vi "Create Sysdef Tree from DB Channel Clusters_RTs_Create MCs.vi"(5 "modeCodes":T4[](array[typedef]), 6 "Autocreate Rx timestamp chans?":bool, 7 "messageBuffers":T2(array[cluster]), 8 "error in (no error)":errorcluster, 10 "rtMode":T3, 11 "Section Ptr in":T1 format="%.0x") -> (0 "error out":errorcluster)   [LabVIEW 2017, in "Ballard 1553 System Explorer.lvlib"]
uses:
  Ballard 1553 System Explorer.lvlib
  <vilib>/NI Veristand/Custom Device API/Custom Device Item Ref.ctl
  Parse XML Ballard/Ballard_RT modeCode.ctl
  Parse XML Ballard/Ballard_RT direction.ctl
  Parse XML Ballard/Ballard_RT rtMode.ctl
  <vilib>/NI Veristand/Custom Device API/Custom Device Channel Type.ctl
  <vilib>/NI Veristand/Custom Device API/Custom Device Channel.ctl
  Shared/Controls and Global/Global.vi
  <vilib>/NI Veristand/Custom Device API/Set Item Property (I32).vi
  <vilib>/NI Veristand/Custom Device API/Set Item Property (U16).vi
  <vilib>/NI VeriStand/Custom Device API/Custom Device API.lvlib
  Shared/Ballard 1553 Shared.lvlib
panel:
  out "Section Ptr out":T1 format="%.0x"
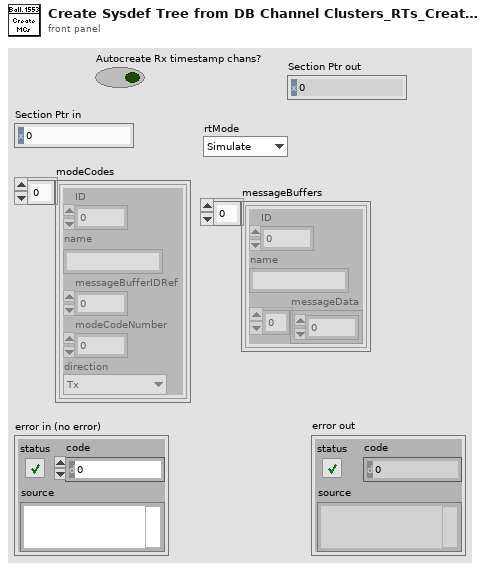
[diagram p1: front panel]
types:
  T1 = typedef "Custom Device API.lvlib/Custom Device Item Ref.ctl" = u64
  T2 = cluster{"ID":i32, "name":string, "messageData":u16[]}[]
  T3 = typedef "Ballard 1553 System Explorer.lvlib/Ballard_RT rtMode.ctl" = enum16{"Simulate", "Monitor", "Disable"}
  T4 = typedef "Ballard 1553 System Explorer.lvlib/Ballard_RT modeCode.ctl" = cluster{"ID":i32, "name":string, "messageBufferIDRef":i32, "modeCodeNumber":i8, "direction":T5}
  T5 = typedef "Ballard 1553 System Explorer.lvlib/Ballard_RT direction.ctl" = enum16{"Tx", "Rx"}
  T6 = typedef "Custom Device API.lvlib/Custom Device Channel Type.ctl" = enum16{"Input", "Output"}
  T7 = typedef "Custom Device API.lvlib/Custom Device Channel.ctl" = cluster{"Type":T6, "Units":string, "Default Value":dbl, "Faultable":bool, "Scalable":bool}
  T8 = enum16{"DW", "STC", "SPC", "SW", "TI MC", "AC", "TI WC"}
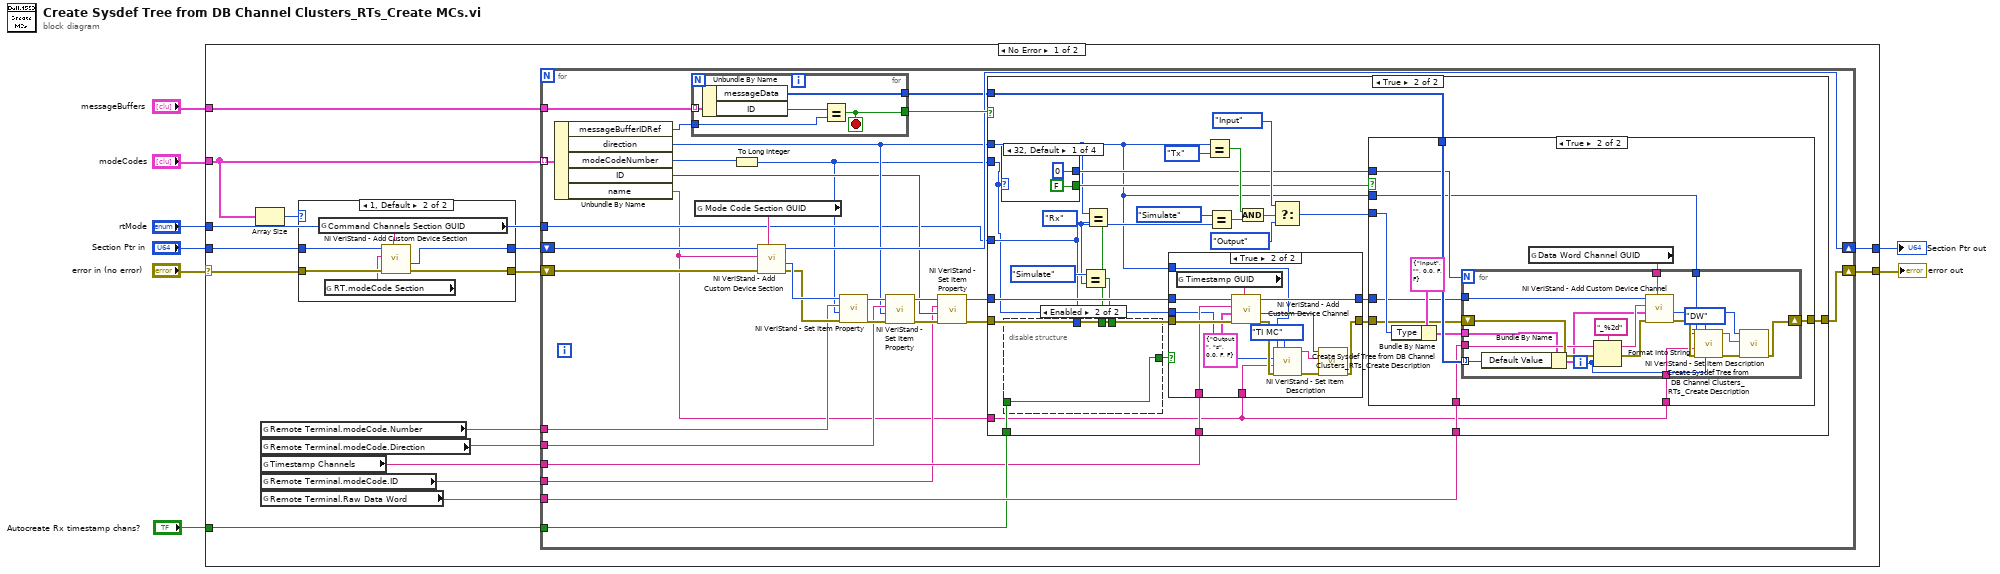
[diagram p0: block diagram]
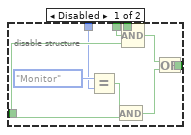
[diagram p3: hidden frame]
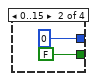
[diagram p4: hidden frame]
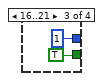
[diagram p5: hidden frame]
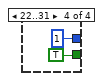
[diagram p6: hidden frame]
diagram:
  n1 = case shown="No Error" "error in (no error)" {
    selector: "error in (no error)" -> [w12 w165]
    tunnel: [w24 w164] -> w8
    tunnel: [w23 w165] -> w2
    tunnel: "modeCodes" -> [w14 _]
    tunnel: "Autocreate Rx timestamp chans?" -> [w21 _]
    tunnel: "messageBuffers" -> [w20 _]
    tunnel: "Section Ptr in" -> [w13 w164]
    tunnel: "rtMode" -> [w16 _]
    frame No Error {
      n2 = Array Size(array=w14) -> (size(s)=w15:i32)
      n3 = global read "Global.vi" "Remote Terminal.modeCode.Number"() -> (w17:string)
      n4 = global read "Global.vi" "Remote Terminal.modeCode.Direction"() -> (w18:string)
      n5 = global read "Global.vi" "Timestamp Channels"() -> (w22:string)
      n6 = global read "Global.vi" "Remote Terminal.modeCode.ID"() -> (w9:string)
      n7 = global read "Global.vi" "Remote Terminal.Raw Data Word"() -> (w19:string)
      n8 = case shown="1, Default" w15 {
        tunnel: w12 -> [w157 w162]
        tunnel: w13 -> [w156 w163]
        tunnel: [w157 w161] -> w10
        tunnel: [w156 w158] -> w11
        frame 0 {
        }
        frame 1, Default {
          n9 = global read "Global.vi" "Command Channels Section GUID"() -> (w160:string)
          n10 = global read "Global.vi" "RT.modeCode Section"() -> (w159:string)
          n11 = call <vilib>:"NI VeriStand - Add Custom Device Section.vi"("GUID (Default Section)"=w160, "error in (no error)"=w162, "Section Name"=w159, "Parent Ref in"=w163) -> ("error out"=w161:errorcluster, "Section Ptr"=w158:T1)  [unwired: 4 in, 2 out]
        }
      }
      n12 = for {
        tunnel: w14 -> [w54] mode=indexing
        shift-right: [w41] -> w23
        shift-left: w10 -> [w27]
        shift-right: [w42] -> w24
        shift-left: w11 -> [w53]
        tunnel: w17 -> [w50]
        tunnel: w18 -> [w47]
        tunnel: w19 -> [w39]
        tunnel: w20 -> [w45]
        tunnel: w21 -> [w38]
        tunnel: w22 -> [w37]
        tunnel: w9 -> [w29]
        tunnel: w16 -> [w28]
        n13 = Unbundle By Name(w54) -> ("messageBufferIDRef"=w44:i32, "direction"=w35:T5, "modeCodeNumber"=w36:i8, "ID"=w30:i32, "name"=w25:string)
        n14 = for {
          tunnel: w45 -> [w155] mode=indexing
          tunnel: w44 -> [w153]
          tunnel: [w152] -> w40
          tunnel: [w151] -> w43
          stop <- w151 stop-if-true
          n15 = Unbundle By Name(w155) -> ("messageData"=w152:u16[], "ID"=w154:i32)
          n16 = Equal?(x=w154, y=w153) -> (x = y?=w151:bool)
        }
        n17 = global read "Global.vi" "Mode Code Section GUID"() -> (w46:string)
        n18 = To Long Integer(number=w36) -> (32bit integer=w26:i32)
        n19 = call <vilib>:"NI VeriStand - Add Custom Device Section.vi"("GUID (Default Section)"=w46, "error in (no error)"=w27, "Section Name"=w25, "Parent Ref in"=w53) -> ("error out"=w51:errorcluster, "Section Ptr"=w52:T1, "Parent Ref out"=w42:T1)  [unwired: 4 in, 1 out]
        n20 = call-poly <vilib>:"NI VeriStand - Set Item Property.vi"("error in (no error)"=w51, "Value"=w26, "Property Name"=w50, "Item Ref in"=w52) -> ("error out"=w49:errorcluster, "Item Ref out"=w48:T1)  [unwired: 5 in, 1 out]
        n21 = call-poly <vilib>:"NI VeriStand - Set Item Property.vi"("error in (no error)"=w49, "Value"=w35, "Property Name"=w47, "Item Ref in"=w48) -> ("error out"=w33:errorcluster, "Item Ref out"=w34:T1)  [unwired: 5 in, 1 out]
        n22 = call-poly <vilib>:"NI VeriStand - Set Item Property.vi"("error in (no error)"=w33, "Value"=w30, "Property Name"=w29, "Item Ref in"=w34) -> ("error out"=w31:errorcluster, "Item Ref out"=w32:T1)  [unwired: 5 in, 1 out]
        n23 = case shown="True" w43 {
          tunnel: w31 -> [w55 w71]
          tunnel: w32 -> [_ w72]
          tunnel: [w55 w73] -> w41
          tunnel: w40 -> [_ w83]
          tunnel: w39 -> [_ w82]
          tunnel: w28 -> [_ w64]
          tunnel: w35 -> [_ w57]
          tunnel: w38 -> [_ w69]
          tunnel: w37 -> [_ w63]
          tunnel: w26 -> [_ w58]
          tunnel: w25 -> [_ w56]
          frame False {
          }
          frame True {
            n24 = case shown="32, Default" w58 {
              tunnel: [i8 0 ("Words (WC)") i8 0 ("Words (WC)") i8 1 ("Words (WC)") i8 1 ("Words (WC)")] -> w59
              tunnel: [FALSE ("2 Status Channels") FALSE ("2 Status Channels") TRUE ("2 Status Channels") TRUE ("2 Status Channels")] -> w60
              frame 32, Default {
              }
              frame 0..15 {
              }
              frame 16..21 {
              }
              frame 22..31 {
              }
            }
            n25 = Equal?(x=Ballard_RT_rtMode."Simulate", y=w64) -> (x = y?=w67:bool)
            n26 = Equal?(x=w57, y=Ballard_RT_direction."Rx") -> (x = y?=w65:bool)
            n27 = disable-structure shown="Enabled" {
              disable-tunnel: [w92 w93] -> w70
              disable-tunnel: w69 -> [w88 w93]
              disable-tunnel: w67 -> [w86 _]
              disable-tunnel: w65 -> [w85 _]
              disable-tunnel: w64 -> [w84 _]
              frame Disabled {
                n28 = Equal?(x=Ballard_RT_rtMode."Monitor", y=w84) -> (x = y?=w90:bool)
                n29 = And(x=w90, y=w88) -> (x .and. y?=w89:bool)
                n30 = Compound Arithmetic op=AND(w86, w85, w88) -> (w87:bool)
                n31 = Or(x=w87, y=w89) -> (x .or. y?=w92:bool)
              }
              frame Enabled {
              }
            }
            n32 = case shown="True" w70 {
              tunnel: w72 -> [w135 w150]
              tunnel: w71 -> [w134 w149]
              tunnel: [w135 w148] -> w61
              tunnel: [w134 w140] -> w62
              tunnel: w63 -> [_ w145]
              tunnel: w56 -> [_ w139]
              tunnel: w57 -> [_ w138]
              tunnel: w58 -> [_ w137]
              frame False {
              }
              frame True {
                n33 = global read "Global.vi" "Timestamp GUID"() -> (w147:string)
                n34 = call <vilib>:"NI VeriStand - Add Custom Device Channel.vi"("GUID (Default Channel)"=w147, "error in (no error)"=w149, "Channel"=T7 {"Type"=enum."Output", "Units"="s", "Default Value"=0.0, "Faultable"=FALSE, "Scalable"=FALSE}, "Channel Name"=w145, "Parent Ref in"=w150) -> ("error out"=w141:errorcluster, "Channel Ref"=w142:T1, "Parent Ref out"=w148:T1)  [unwired: 3 in, 1 out]
                n35 = call "Create Sysdef Tree from DB Channel Clusters_RTs_Create Description.vi"("Type"=T8."TI MC", "error in (no error)"=w141, "Name"=w139, "SA/MC"=w137, "Direction"=w138) -> ("error out"=w143:errorcluster, "Description (Out)"=w144:string)  [unwired: 5 in]
                n36 = call <vilib>:"NI VeriStand - Set Item Description.vi"("error in (no error)"=w143, "Description"=w144, "Item Ref in"=w142) -> ("error out"=w140:errorcluster)  [unwired: 6 in, 2 out]
              }
            }
            n37 = Equal?(x=w57, y=Ballard_RT_direction."Tx") -> (x = y?=w78:bool)
            n38 = Equal?(x=Ballard_RT_rtMode."Simulate", y=w64) -> (x = y?=w80:bool)
            n39 = And(x=w78, y=w80) -> (x .and. y?=w77:bool)
            n40 = Select(t=Custom_Device_Channel_Type."Input" ("Type"), s=w77, f=Custom_Device_Channel_Type."Output") -> (s? t:f=w75:T6)
            n41 = case shown="True" w60 {
              tunnel: w83 -> [_ w113]
              tunnel: w82 -> [_ w112]
              tunnel: w75 -> [_ w109]
              tunnel: [w102 w108] -> w73
              tunnel: w62 -> [w102 w107]
              tunnel: w61 -> [_ w106]
              tunnel: w59 -> [_ w105]
              tunnel: w57 -> [_ w104]
              tunnel: w56 -> [_ w103]
              frame False {
              }
              frame True {
                n42 = Bundle By Name(cluster=T7 {"Type"=enum."Input", "Units"="", "Default Value"=0.0, "Faultable"=FALSE, "Scalable"=FALSE} ("Channel"), "Type"=w109) -> (w110:T7)
                n43 = global read "Global.vi" "Data Word Channel GUID"() -> (w114:string)
                n44 = for {
                  N: w105 -> [_]
                  tunnel: w106 -> [w133]
                  tunnel: w112 -> [w126]
                  shift-right: [w121] -> w108
                  shift-left: w107 -> [w131]
                  tunnel: w113 -> [w128] mode=indexing
                  tunnel: w114 -> [w127]
                  tunnel: w110 -> [w125]
                  tunnel: w104 -> [w117]
                  tunnel: w103 -> [w115]
                  i -> [w118]
                  n45 = Bundle By Name(cluster=w125, "Default Value"=w128) -> (w124:T7)
                  n46 = Format Into String(format string="_%2d", initial string=w126, error in=w131, w118) -> (resulting string=w129:string, error out=w130:errorcluster)
                  n47 = call <vilib>:"NI VeriStand - Add Custom Device Channel.vi"("GUID (Default Channel)"=w127, "error in (no error)"=w130, "Channel"=w124, "Channel Name"=w129, "Parent Ref in"=w133) -> ("error out"=w122:errorcluster, "Channel Ref"=w119:T1)  [unwired: 3 in, 2 out]
                  n48 = call "Create Sysdef Tree from DB Channel Clusters_RTs_Create Description.vi"("Word Index"=w118, "Type"=T8."DW", "error in (no error)"=w122, "Name"=w115, "Direction"=w117) -> ("error out"=w120:errorcluster, "Description (Out)"=w123:string)  [unwired: 5 in]
                  n49 = call <vilib>:"NI VeriStand - Set Item Description.vi"("error in (no error)"=w120, "Description"=w123, "Item Ref in"=w119) -> ("error out"=w121:errorcluster)  [unwired: 6 in, 2 out]
                }
              }
            }
          }
        }
      }
    }
    frame Error {
    }
  }
  "error out" <- w2
  "Section Ptr out" <- w8
